vi "Berekenen-c.vi"(9 "K":dbl, 10 "Td":dbl, 11 "T":dbl) -> (2 "C":dbl)   [LabVIEW 2021]
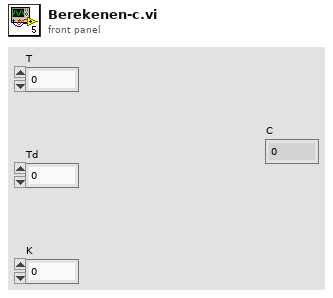
[diagram p1: front panel]
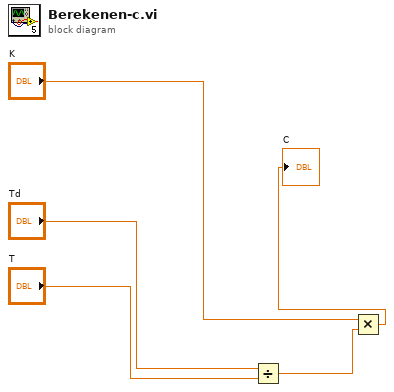
[diagram p0: block diagram]
diagram:
  n1 = Divide(x="Td", y="T") -> (x/y=w4:dbl)
  n2 = Multiply(x="K", y=w4) -> (x*y=→"C":dbl)
